vi "Replase ALR_block.vi"(9 "ALR_block":bool, 10 "N":i32, 11 "ALR_ON_OFF in":T1) -> (3 "ALR_ON_OFF out":T1)   [LabVIEW 2019, in "Alarms.lvlib"]
uses:
  Alarms.lvlib
  Ctl/ALR_ON_OFF.ctl
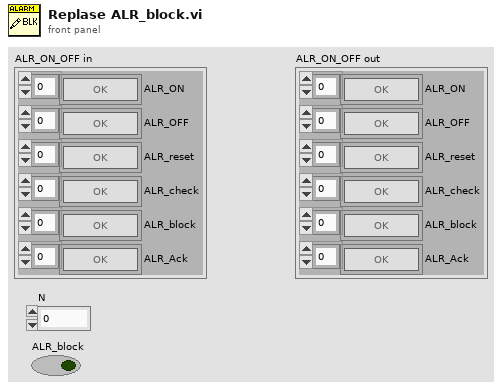
[diagram p1: front panel]
types:
  T1 = typedef "Alarms.lvlib/ALR_ON_OFF.ctl" = cluster{"ALR_ON":bool[], "ALR_OFF":bool[], "ALR_reset":bool[], "ALR_check":bool[], "ALR_block":bool[], "ALR_Ack":bool[]}
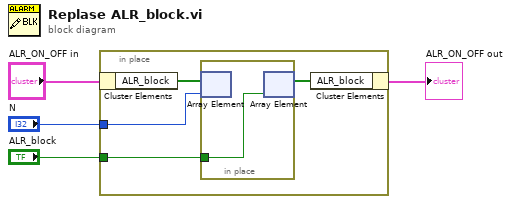
[diagram p0: block diagram]
diagram:
  n1 = in-place {
    in-place-border: "ALR_block" -> [w8]
    in-place-border: "N" -> [w5]
    n2 = in-place-cluster #1("ALR_ON_OFF in") -> ("ALR_block"=w7:bool[])
    n3 = in-place {
      in-place-border: w8 -> [w9]
      n4 = in-place-array #2(w7, w5) -> ()  [unwired: 1 out]
      n5 = in-place-array #2(w9) -> (w6:bool[])  [unwired: 1 out]
    }
    n6 = in-place-cluster #1("ALR_block"=w6) -> (→"ALR_ON_OFF out":T1)
  }
